vi "CRYDate time filename format.vi"() -> (2 "Time string":string, 3 "Date string":string)   [LabVIEW 2013]
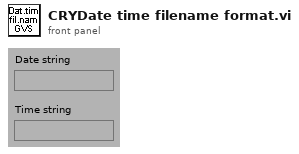
[diagram p1: front panel]
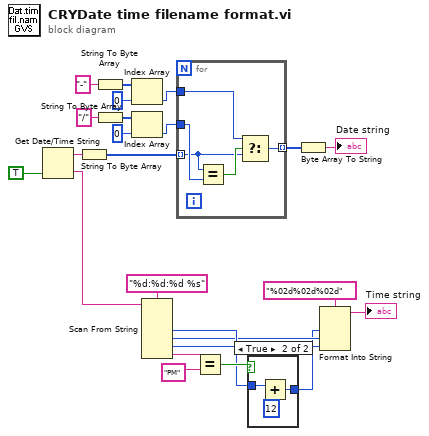
[diagram p0: block diagram]
diagram:
  n1 = Get Date/Time String(want seconds? (F)=TRUE) -> (date string=w23:string, time string=w10:string)  [unwired: 2 in]
  n2 = String To Byte Array(string=w23) -> (unsigned byte array=w19:u8[])
  n3 = String To Byte Array(string="-") -> (unsigned byte array=w18:u8[])
  n4 = String To Byte Array(string="/") -> (unsigned byte array=w21:u8[])
  n5 = Index Array(array=w18, index=0) -> (element=w15:u8)
  n6 = Index Array(array=w21, index=0) -> (element=w20:u8)
  n7 = Scan From String(format string="%d:%d:%d %s", input string=w10) -> (output 1=w6:i32, output 2=w5:i32, output 3=w4:i32, output 4=w9:string)  [unwired: 6 in, 3 out]
  n8 = for {
    tunnel: w20 -> [w29]
    tunnel: w19 -> [w26] mode=indexing
    tunnel: w15 -> [w27]
    tunnel: [w25] -> w14 mode=indexing
    n9 = Equal?(x=w26, y=w29) -> (x = y?=w28:bool)
    n10 = Select(t=w27, s=w28, f=w26) -> (s? t:f=w25:u8)
  }
  n11 = Equal?(x=w9, y="PM") -> (x = y?=w7:bool)
  n12 = case shown="True" w7 {
    tunnel: w6 -> [w30 w33]
    tunnel: [w30 w31] -> w3
    frame False {
    }
    frame True {
      n13 = Add(x=w33, y=12) -> (x+y=w31:i32)
    }
  }
  n14 = Byte Array To String(unsigned byte array=w14) -> (string=→"Date string":string)
  n15 = Format Into String(format string="%02d%02d%02d", w3, w5, w4) -> (resulting string=→"Time string":string)  [unwired: 2 in, 1 out]
